vi "FPGA_Ops_subVI.vi"(8 "error in (no error)":errorcluster, 9 "Chirp":fxp<+,16,3>[](array[numeric]), 10 "Samples to Read":dbl, 11 "FPGA VI Reference Out":refnum<k20>) -> (0 "error out":errorcluster, 1 "Data B":fxp<+,16,3>[](array[numeric]), 2 "Data A":fxp<+,16,3>[](array[numeric]), 3 "Refnum out":refnum<k20>)   [LabVIEW 2017]
doc: "Start and shut down the FPGA program."
uses:
  <vilib>/Utility/error.llb/Error Cluster From Error Code.vi
  <vilib>/rvi/errors/niLvFpgaAdjustHostInterfaceError.vi
  <vilib>/FPGAPlugInAG/Dynamic/niLvFpga_Run_Dynamic.vi
  <vilib>/rvi/interface/nirviMethod/nirviMethod.xnode
  <vilib>/rvi/interface/nirviReadWriteControl/nirviReadWriteControl.xnode
  <vilib>/FPGAPlugInAG/Dynamic/niLvFpga_StartFifo_Dynamic.vi
  <vilib>/rvi/errors/niLvFpgaMergeErrorWithErrorCode.vi
  <vilib>/FPGAPlugInAG/Dynamic/niLvFpga_WriteFifo_Dynamic.vi
  NiFpgaLv.dll
  <vilib>/rvi/interface/Simulation/niFpgaSimulationCallBeginRW.vi
  <vilib>/FPGAPlugInAG/Dynamic/niLvFpga_ReadFifo_Dynamic.vi
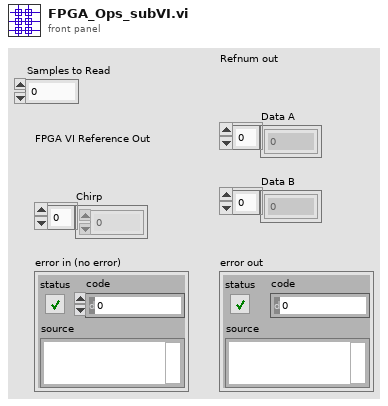
[diagram p1: front panel]
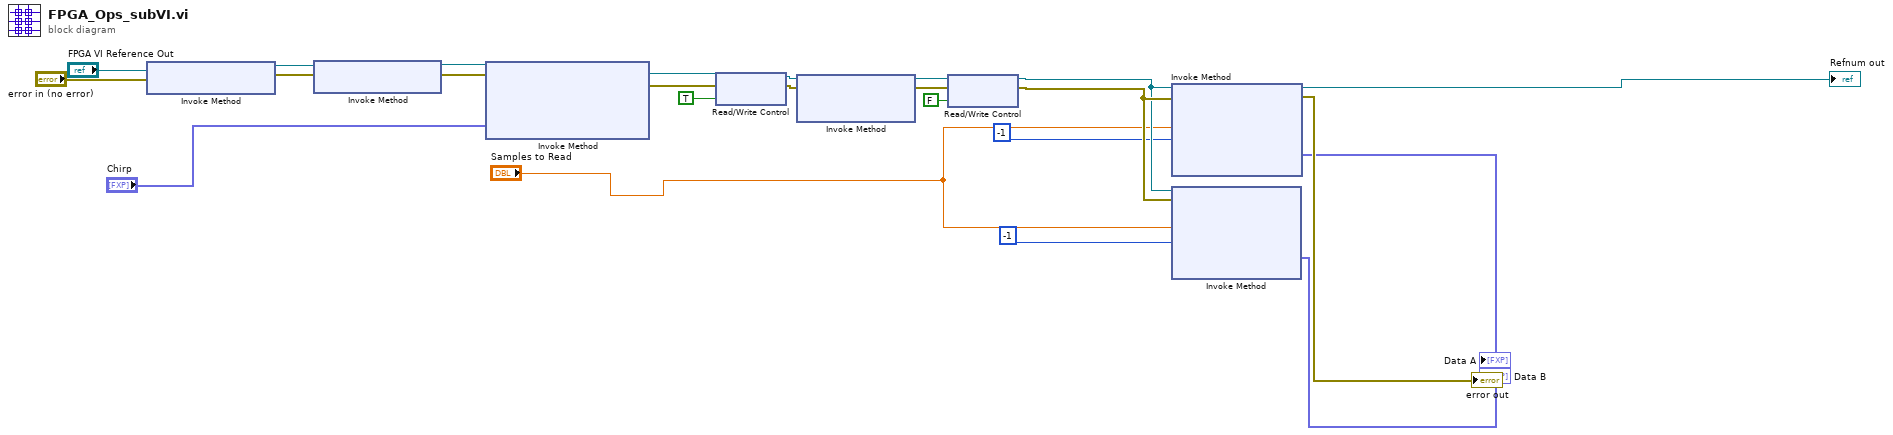
[diagram p0: block diagram]
diagram:
  n1 = xnode "Invoke Method"("FPGA VI Reference In"="FPGA VI Reference Out", "error in"="error in (no error)") -> ("FPGA VI Reference Out"=w13:refnum<k20>, "error out"=w14:errorcluster)
  n2 = xnode "Invoke Method"("FPGA VI Reference In"=w13, "error in"=w14) -> ("FPGA VI Reference Out"=w23:refnum<k20>, "error out"=w24:errorcluster)
  n3 = xnode "Invoke Method"("FPGA VI Reference In"=w23, "error in"=w24, "Data"="Chirp") -> ("FPGA VI Reference Out"=w9:refnum<k20>, "error out"=w10:errorcluster)  [unwired: 1 in, 1 out]
  n4 = xnode "Read/Write Control"("FPGA VI Reference In"=w9, "error in"=w10, "Wavegen!"=TRUE) -> ("FPGA VI Reference Out"=w11:refnum<k20>, "error out"=w12:errorcluster)
  n5 = xnode "Invoke Method"("FPGA VI Reference In"=w11, "error in"=w12) -> ("FPGA VI Reference Out"=w18:refnum<k20>, "error out"=w19:errorcluster)  [unwired: 1 in]
  n6 = xnode "Read/Write Control"("FPGA VI Reference In"=w18, "error in"=w19, "Wavegen!"=FALSE) -> ("FPGA VI Reference Out"=w21:refnum<k20>, "error out"=w22:errorcluster)
  n7 = xnode "Invoke Method"("FPGA VI Reference In"=w21, "error in"=w22, "Number of Elements"="Samples to Read", "Timeout (ms)"=-1) -> ("FPGA VI Reference Out"=→"Refnum out":refnum<k20>, "error out"=→"error out":errorcluster, "Data"=→"Data A":fxp<+,16,3>[])  [unwired: 1 out]
  n8 = xnode "Invoke Method"("FPGA VI Reference In"=w21, "error in"=w22, "Number of Elements"="Samples to Read", "Timeout (ms)"=-1) -> ("Data"=→"Data B":fxp<+,16,3>[])  [unwired: 3 out]
